vi "5492_AutonomousTurnTuning.vi"(8 "error in (no error)":errorcluster, 10 "Turn Type":string="Numeric") -> (0 "error out (no error)":errorcluster)   [LabVIEW 2017]
uses:
  <vilib>/Rock Robotics/WPI/ThirdParty/Cross The Road Electronics/Phoenix-LabVIEW/Motor Controller/Controls/CTRE_Phoenix_MotorControl_ControlMode.ctl
  <vilib>/Rock Robotics/WPI/Utilities/WPI_GetSetVariantRefNum.vi
  <vilib>/Rock Robotics/Network Tables/NT Read Number.vi
  <vilib>/Rock Robotics/WPI/RobotDrive/WPI_RobotDriveSafetyCheck.vi
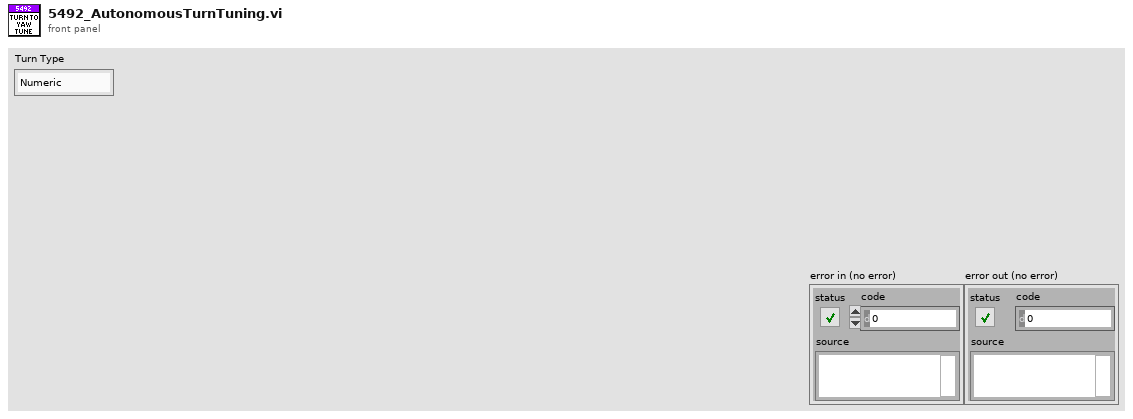
[diagram p1: front panel]
types:
  T1 = typedef "CTRE_Phoenix_MotorControl_ControlMode.ctl" = u16
  T2 = cluster{"Yaw":dbl, "Roll":dbl, "Pitch":dbl, "Heading":dbl, "Fused Heading":dbl}
  T3 = typedef "WPI_RobotDriveDevRef.ctl" = cluster{"DevStatus":errorcluster, "Motors[]":T4[], "Square Inputs":bool, "Max Output":dbl}
  T4 = typedef "WPI_MotorControlDeviceRef.ctl" = cluster{"DeviceStatus":errorcluster, "Type":T5, "PWM":cluster{"PWM Channel":T6, "DeadBand":T7}, "CAN":cluster{"Device Number":u8, "SetOutput VI Ref":variant, "GetOutput VI Ref":variant, "Enable VI Ref":variant, "Disable VI Ref":variant, "Data":variant}, "Invert":bool, "DIO PWM":cluster{"PWM \"Enable\" Channel":T6, "DIOChannel":T8, "PWM Rate":dbl}}
  T5 = typedef "WPI_MotorControlType.ctl" = enum16{"PWM", "CAN", "DIO PWM"}
  T6 = typedef "FPGA_DIOPWMChannel.ctl" = enum8{"PWM 0", "PWM 1", "PWM 2", "PWM 3", "PWM 4", "PWM 5", "PWM 6", "PWM 7", "PWM 8", "PWM 9", "PWM MXP 0", "PWM MXP 1", "PWM MXP 2", "PWM MXP 3", "PWM MXP 4", "PWM MXP 5", "PWM MXP 6", "PWM MXP 7", "PWM MXP 8", "PWM MXP 9", "Invalid"}
  T7 = typedef "WPI_PWMDeadband.ctl" = cluster{"Name":string, "maxPositivePwm":i32, "minPositivePwm":i32, "centerPwm":i32, "maxNegativePwm":i32, "minNegativePwm":i32, "angularRange":u16}
  T8 = typedef "FPGA_DIOChannel.ctl" = enum8{"DIO 0", "DIO 1", "DIO 2", "DIO 3", "DIO 4", "DIO 5", "DIO 6", "DIO 7", "DIO 8", "DIO 9", "DIO MXP 0", "DIO MXP 1", "DIO MXP 2", "DIO MXP 3", "DIO MXP 4", "DIO MXP 5", "DIO MXP 6", "DIO MXP 7", "DIO MXP 8", "DIO MXP 9", "DIO MXP 10", "DIO MXP 11", "DIO MXP 12", "DIO MXP 13", "DIO MXP 14", "DIO MXP 15", "SPI Port CS1", "SPI Port CS2", "SPI Port CS3", "SPI Port MISO", "SPI Port MOSI", "Invalid"}
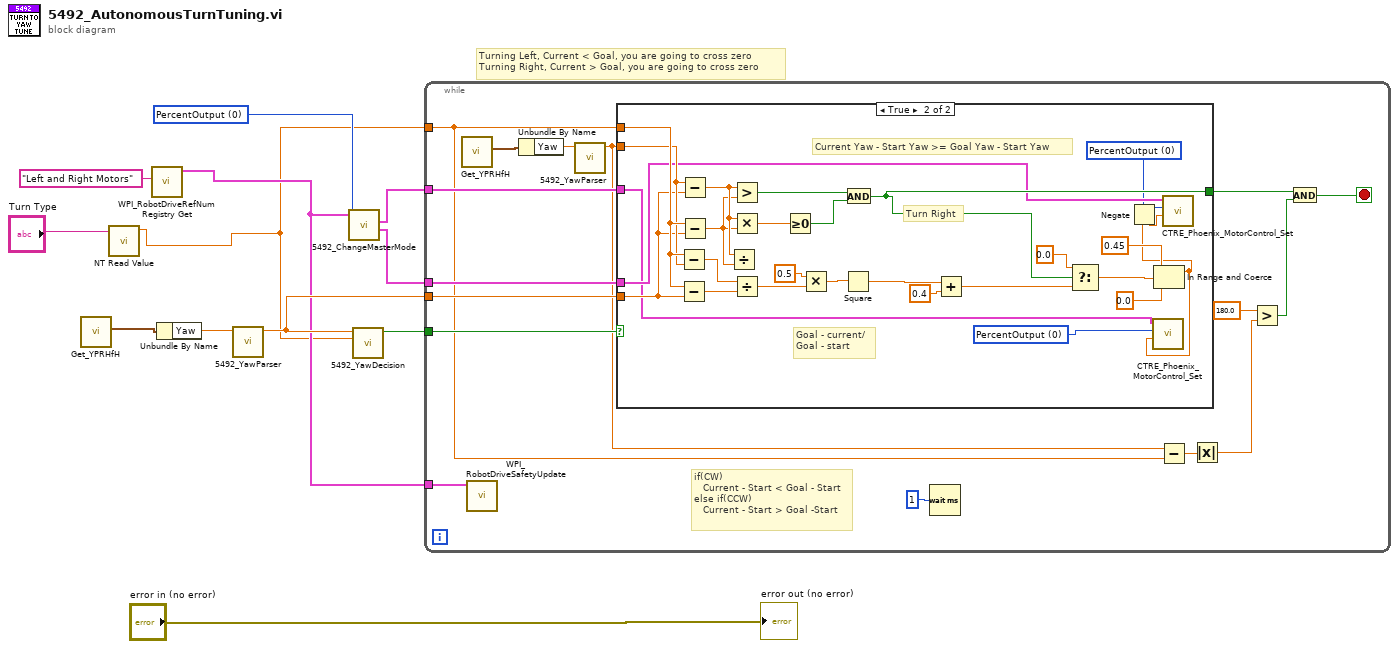
[diagram p0: block diagram]
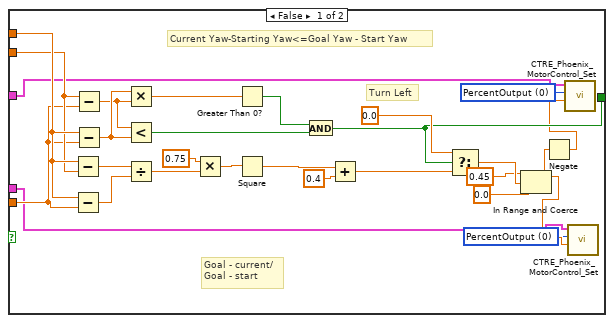
[diagram p2: hidden frame]
diagram:
  w5 = T1 0 items=["PercentOutput"=0, "Position"=1, "Velocity"=2, "Current"=3, "Follower"=5, "MotionProfile"=6, "MotionMagic"=7, "MotionMagicArc"=8, "MotionProfileArc"=10, "Disabled"=15] ("Control Mode")
  # "Turning Left, Current < Goal, you are going to cross zero\nTurning Right, Current > Goal, you are going to cross zero"
  n1 = call <vilib>:"Get_YPRHfH.vi"() -> ("YRPHfH"=w6:T2)  [unwired: 11 in]
  n2 = call-poly <vilib>:"NT Read Value.vi"("Name"="Turn Type") -> ("Numeric"=w2:dbl)  [unwired: 9 in, 1 out]
  n3 = call <vilib>:"WPI_RobotDriveRefNum Registry Get.vi"("refnum name"="Left and Right Motors") -> ("RobotDriveDevRef"=w3:T3)  [unwired: 9 in, 1 out]
  n4 = Unbundle By Name(w6) -> ("Yaw"=w10:dbl)
  n5 = call "5492_YawParser.vi"("Yaw"=w10) -> ("Parsed Yaw"=w8:dbl)  [unwired: 10 in]
  n6 = call "5492_ChangeMasterMode.vi"("Control Mode"=w5, "RobotDriveDevRef"=w3) -> ("CAN Talon SRX Right"=w11:T4, "CAN Talon SRX Ref Left"=w12:T4)  [unwired: 7 in, 1 out]
  n7 = call "5492_YawDecision.vi"("Yaw Goallll"=w2, "Parsed Yaw"=w8) -> ("Right???"=w9:bool)  [unwired: 9 in]
  n8 = while {
    tunnel: w12 -> [w27]
    tunnel: w11 -> [w26]
    tunnel: w9 -> [w25]
    tunnel: w8 -> [w23]
    tunnel: w2 -> [w20]
    tunnel: w3 -> [w13]
    stop <- w14 stop-if-true
    # "if(CW)\n   Current - Start < Goal - Start\nelse if(CCW)\n   Current - Start > Goal -Start"
    n9 = call <vilib>:"Get_YPRHfH.vi"() -> ("YRPHfH"=w22:T2)  [unwired: 11 in]
    n10 = call <vilib>:"WPI_RobotDriveSafetyUpdate.vi"("RobotDriveDevRef"=w13) -> ()  [unwired: 1 in, 10 out]
    n11 = Unbundle By Name(w22) -> ("Yaw"=w24:dbl)
    n12 = call "5492_YawParser.vi"("Yaw"=w24) -> ("Parsed Yaw"=w21:dbl)  [unwired: 10 in]
    n13 = case shown="True" w25 {
      tunnel: w27 -> [w34 w56]
      tunnel: w26 -> [w31 w61]
      tunnel: w21 -> [w40 w68]
      tunnel: w23 -> [w39 w67]
      tunnel: w20 -> [w41 w75]
      tunnel: [w54 w80] -> w15
      frame False {
        w29 = T1 0 items=["PercentOutput"=0, "Position"=1, "Velocity"=2, "Current"=3, "Follower"=5, "MotionProfile"=6, "MotionMagic"=7, "MotionMagicArc"=8, "MotionProfileArc"=10, "Disabled"=15] ("Control Mode")
        w32 = T1 0 items=["PercentOutput"=0, "Position"=1, "Velocity"=2, "Current"=3, "Follower"=5, "MotionProfile"=6, "MotionMagic"=7, "MotionMagicArc"=8, "MotionProfileArc"=10, "Disabled"=15] ("Control Mode")
        # "Current Yaw-Starting Yaw<=Goal Yaw - Start Yaw"
        # "Goal - current/\nGoal - start"
        # "Turn Left"
        n14 = Subtract(x=w41, y=w40) -> (x-y=w42:dbl)
        n15 = Subtract(x=w41, y=w39) -> (x-y=w43:dbl)
        n16 = Subtract(x=w40, y=w39) -> (x-y=w51:dbl)
        n17 = Subtract(x=w41, y=w39) -> (x-y=w52:dbl)
        n18 = Multiply(x=w52, y=w51) -> (x*y=w50:dbl)
        n19 = Less?(x=w51, y=w52) -> (x < y?=w53:bool)
        n20 = Divide(x=w42, y=w43) -> (x/y=w46:dbl)
        n21 = Multiply(x=0.75, y=w46) -> (x*y=w45:dbl)
        n22 = Greater Than 0?(x=w50) -> (x > 0?=w49:bool)
        n23 = Square(x=w45) -> (x^2=w44:dbl)
        n24 = And(x=w49, y=w53) -> (x .and. y?=w54:bool)
        n25 = Add(x=w44, y=0.4) -> (x+y=w38:dbl)
        n26 = Select(t=0.0, s=w54, f=w38) -> (s? t:f=w37:dbl)
        n27 = In Range and Coerce(upper limit=0.45, x=w37, lower limit=0.0) -> (coerced(x)=w30:dbl)  [unwired: 1 out]
        n28 = Negate(x=w30) -> (-x=w33:dbl)
        n29 = call <vilib>:"CTRE_Phoenix_MotorControl_Set.vi"("Output"=w33, "Control Mode"=w32, "PhoenixMotorControlDevRef"=w34) -> ()  [unwired: 7 in, 2 out]
        n30 = call <vilib>:"CTRE_Phoenix_MotorControl_Set.vi"("Output"=w30, "Control Mode"=w29, "PhoenixMotorControlDevRef"=w31) -> ()  [unwired: 7 in, 2 out]
      }
      frame True {
        w58 = T1 0 items=["PercentOutput"=0, "Position"=1, "Velocity"=2, "Current"=3, "Follower"=5, "MotionProfile"=6, "MotionMagic"=7, "MotionMagicArc"=8, "MotionProfileArc"=10, "Disabled"=15] ("Control Mode")
        w59 = T1 0 items=["PercentOutput"=0, "Position"=1, "Velocity"=2, "Current"=3, "Follower"=5, "MotionProfile"=6, "MotionMagic"=7, "MotionMagicArc"=8, "MotionProfileArc"=10, "Disabled"=15] ("Control Mode")
        # "Current Yaw - Start Yaw >= Goal Yaw - Start Yaw"
        # "Goal - current/\nGoal - start"
        # "Turn Right"
        n31 = Subtract(x=w75, y=w68) -> (x-y=w74:dbl)
        n32 = Subtract(x=w75, y=w67) -> (x-y=w73:dbl)
        n33 = Subtract(x=w68, y=w67) -> (x-y=w77:dbl)
        n34 = Subtract(x=w75, y=w67) -> (x-y=w76:dbl)
        n35 = Divide(x=w77, y=w76) -> ()  [unwired: 1 out]
        n36 = Greater?(x=w77, y=w76) -> (0:w81:bool)
        n37 = Multiply(x=w77, y=w76) -> (x*y=w79:dbl)
        n38 = Divide(x=w74, y=w73) -> (x/y=w70:dbl)
        n39 = Greater Or Equal To 0?(x=w79) -> (x >= 0?=w78:bool)
        n40 = Multiply(x=0.5, y=w70) -> (x*y=w71:dbl)
        n41 = Square(x=w71) -> (x^2=w72:dbl)
        n42 = And(x=w81, y=w78) -> (x .and. y?=w80:bool)
        n43 = Add(x=w72, y=0.4) -> (x+y=w65:dbl)
        n44 = Select(t=0.0, s=w80, f=w65) -> (s? t:f=w63:dbl)
        n45 = In Range and Coerce(upper limit=0.45, x=w63, lower limit=0.0) -> (coerced(x)=w57:dbl)  [unwired: 1 out]
        n46 = Negate(x=w57) -> (-x=w60:dbl)
        n47 = call <vilib>:"CTRE_Phoenix_MotorControl_Set.vi"("Output"=w57, "Control Mode"=w58, "PhoenixMotorControlDevRef"=w56) -> ()  [unwired: 7 in, 2 out]
        n48 = call <vilib>:"CTRE_Phoenix_MotorControl_Set.vi"("Output"=w60, "Control Mode"=w59, "PhoenixMotorControlDevRef"=w61) -> ()  [unwired: 7 in, 2 out]
      }
    }
    n49 = Wait (ms)(milliseconds to wait=u32 1) -> ()  [unwired: 1 out]
    n50 = Subtract(x=w21, y=w20) -> (x-y=w19:dbl)
    n51 = Absolute Value(x=w19) -> (abs(x)=w18:dbl)
    n52 = Greater?(x=180.0, y=w18) -> (0:w16:bool)
    n53 = And(x=w15, y=w16) -> (x .and. y?=w14:bool)
  }
  "error out (no error)" <- "error in (no error)"
